vi "Init Gyro.vi"(8 "error in (no error)":errorcluster) -> (0 "error out":errorcluster, 1 "Gyro Bias":cluster{"X":dbl, "Y":dbl, "Z":dbl}, 3 "I2C Ref Out":T1)   [LabVIEW 2017]
uses:
  <vilib>/myRIO/Instrument Drivers/Onboard IO/I2C/typedefs/I2C Reference.ctl
  <vilib>/myRIO/Common/Instrument Driver Framework/Utilities/typedefs/myRIO Generic Hardware Reference.ctl
  <vilib>/myRIO/Common/Instrument Driver Framework/Utilities/typedefs/Hardware Version Enum.ctl
  <vilib>/myRIO/Common/Instrument Driver Framework/Utilities/typedefs/myRIO v1.0 Reference.ctl
  <vilib>/myRIO/Common/Instrument Driver Framework/Utilities/typedefs/Generic FPGA Reference.ctl
  <vilib>/myRIO/Common/Instrument Driver Framework/myRIO v1.0/I2C/typedefs/I2C Channels Enum.ctl
  <vilib>/myRIO/Instrument Drivers/Onboard IO/I2C/typedefs/I2C Configuration.ctl
  <vilib>/myRIO/Instrument Drivers/Onboard IO/I2C/typedefs/I2C Transfer Rate.ctl
  <vilib>/userdefined/High Color/nirio_resource_hc.ctl
  MPU6050 Private class data.vi
  <vilib>/myRIO/Instrument Drivers/Onboard IO/I2C/I2C.lvlib
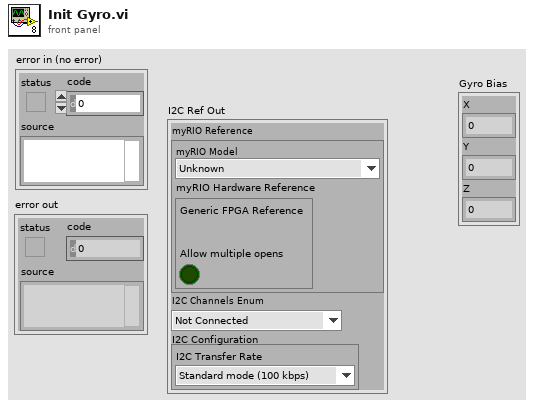
[diagram p1: front panel]
types:
  T1 = typedef "I2C.lvlib/I2C Reference.ctl" = cluster{"myRIO Reference":T2, "I2C Channels Enum":T6, "I2C Configuration":T7}
  T2 = typedef "myRIO Generic Hardware Reference.ctl" = cluster{"myRIO Model":T3, "myRIO Hardware Reference":T4}
  T3 = typedef "Hardware Version Enum.ctl" = enum16{"Unknown", "myRIO-1900", "myRIO-1950", "roboRIO", "NI ELVIS RIO CM"}
  T4 = typedef "myRIO v1.0 Reference.ctl" = cluster{"Generic FPGA Reference":T5, "Allow multiple opens":bool}
  T5 = typedef "Generic FPGA Reference.ctl" = refnum<k20>
  T6 = typedef "I2C Channels Enum.ctl" = enum16{"Not Connected", "A/I2C", "B/I2C", "I2C/I2C"}
  T7 = typedef "I2C.lvlib/I2C Configuration.ctl" = cluster{"I2C Transfer Rate":T8}
  T8 = typedef "I2C.lvlib/I2C Transfer Rate.ctl" = enum16{"Standard mode (100 kbps)", "Fast mode (400 kbps)"}
  T9 = typedef "nirio_resource_hc.ctl" = tag
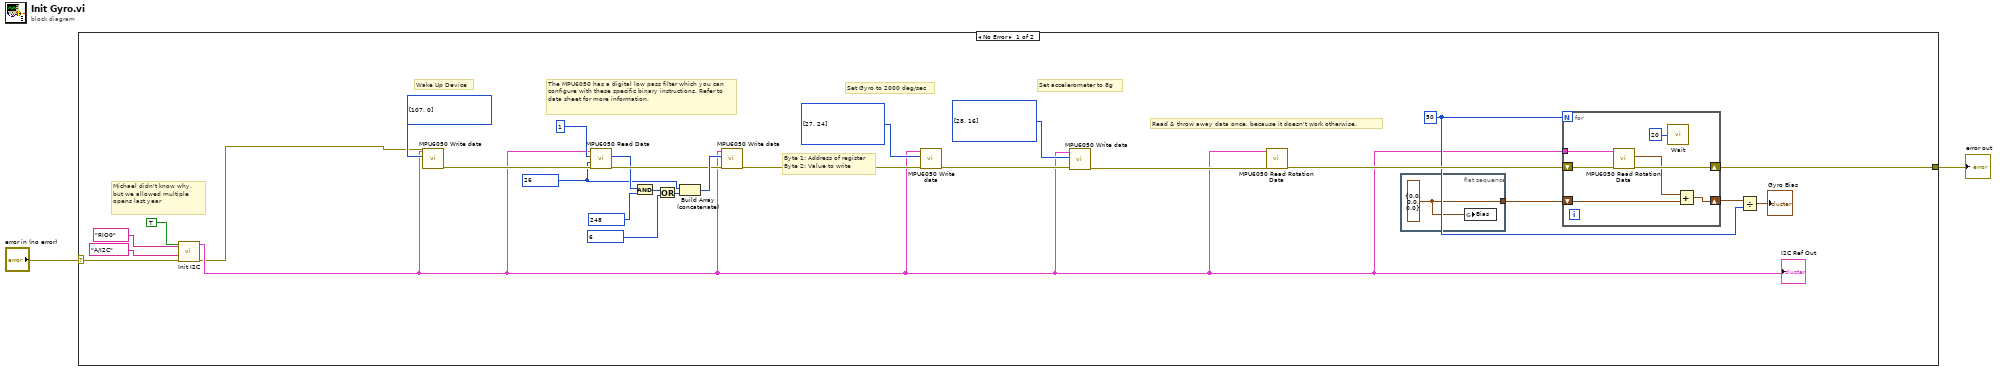
[diagram p0: block diagram]
diagram:
  n1 = case shown="No Error" "error in (no error)" {
    selector: "error in (no error)" -> [w30 w39]
    tunnel: [w29 w39] -> w1
    frame No Error {
      w14 = u8 26
      w26 = 50
      # "Byte 1: Address of register\nByte 2: Value to write"
      # "Set accelerometer to 8g"
      # "Michael didn't know why, but we allowed multiple opens last year"
      # "Wake Up Device"
      # "The MPU6050 has a digital low pass filter which you can configure with these specific binary instructions. Refer to data sheet for more information."
      # "Set Gyro to 2000 deg/sec"
      # "Read & throw away data once, because it doesn't work otherwise."
      n2 = call "Init I2C.vi"("error in"=w30, "Channel Name"=tag "A/I2C", "Resource name"=T9 "RIO0", "Allow multiple opens?"=TRUE) -> ("error out"=w3:errorcluster, "I2C Ref Out"=w4:T1)  [unwired: 6 in]
      "I2C Ref Out" <- w4
      n3 = call "MPU6050 Write data.vi"("I2C Ref In"=w4, "Bytes to Write"=u8[] [107, 0], "error in (no error)"=w3) -> ("error out"=w17:errorcluster)  [unwired: 7 in]
      n4 = call "MPU6050 Read Data.vi"("error in (no error)"=w17, "Start Address"=w14, "Data Length"=u8 1, "I2C Ref In"=w4) -> ("error out"=w18:errorcluster, "Data read"=w15:u8[])  [unwired: 6 in]
      n5 = And(x=w15, y=u8 248) -> (x .and. y?=w21:u8[])
      n6 = Or(x=w21, y=u8 6) -> (x .or. y?=w22:u8[])
      n7 = Build Array (concatenate)(w14, w22) -> (w19:u8[])
      n8 = call "MPU6050 Write data.vi"("I2C Ref In"=w4, "Bytes to Write"=w19, "error in (no error)"=w18) -> ("error out"=w25:errorcluster)  [unwired: 7 in]
      n9 = call "MPU6050 Write data.vi"("I2C Ref In"=w4, "Bytes to Write"=u8[] [27, 24], "error in (no error)"=w25) -> ("error out"=w9:errorcluster)  [unwired: 7 in]
      n10 = call "MPU6050 Write data.vi"("I2C Ref In"=w4, "Bytes to Write"=u8[] [28, 16], "error in (no error)"=w9) -> ("error out"=w8:errorcluster)  [unwired: 7 in]
      n11 = call "MPU6050 Read Rotation Data.vi"("error in (no error)"=w8, "I2C Ref In"=w4) -> ("error out"=w28:errorcluster)  [unwired: 7 in, 2 out]
      n12 = flat-sequence {
        tunnel: [w31] -> w11
        frame #0 {
          w31 = cluster{"X":dbl, "Y":dbl, "Z":dbl} {"X"=0.0, "Y"=0.0, "Z"=0.0} ("Gyro Data")
          n13 = global write "MPU6050 Private class data.vi" "Bias"(w31) -> ()
        }
      }
      n14 = for {
        N: w26 -> [_]
        shift-right: [w37] -> w29
        shift-left: w28 -> [w38]
        shift-right: [w36] -> w27
        shift-left: w11 -> [w34]
        tunnel: w4 -> [w32]
        n15 = call "MPU6050 Read Rotation Data.vi"("error in (no error)"=w38, "I2C Ref In"=w32) -> ("error out"=w37:errorcluster, "rad/s"=w35:cluster{"X":dbl, "Y":dbl, "Z":dbl})  [unwired: 7 in, 1 out]
        n16 = call "Wait"("Count(mSec)"=u32 20 ("Count(uSec)")) -> ()  [unwired: 1 out]
        n17 = Add(x=w35, y=w34) -> (x+y=w36:cluster{"X":dbl, "Y":dbl, "Z":dbl})
      }
      n18 = Divide(x=w27, y=w26) -> (x/y=→"Gyro Bias":cluster{"X":dbl, "Y":dbl, "Z":dbl})
    }
    frame Error {
    }
  }
  "error out" <- w1
